vi "FPGA_balancing_noGPS.vi"() -> ()   [LabVIEW 2019]
uses:
  <vilib>/rvi/Emulation/niFpgaGetClockAttributes.vi
  <vilib>/rvi/Emulation/niFpgaSctlEmulationGetInTimedLoop.vi
  <vilib>/rvi/Emulation/niFpgaEmulationReportErrorSimple.vi
  <vilib>/rvi/eio/common/nirviEmuTemplateMethod_errors.vi
  <vilib>/rvi/Emulation/niFpgaCriticalErrorInLSC.vi
  Sub VIs/GlobalVariables.vi
  <vilib>/rvi/Emulation/niFpgaProcessEmulError.vi
  <vilib>/eio/EIONode/EIONode.xnode
  Sub VIs/GPS/UART 8N1/UART 8N1 (FPGA).lvlib
panel:
  out "ESTOP":bool
  in  "Hall Edge Detection":enum16{"falling", "rising"}(ring)
  out "Steering Current":u16
  in  "Steering Enable":bool
  out "SPI Read Acc Data":u8[](array[numeric])
  out "SPI Read Gyro Data":u8[](array[numeric])
  out "Encoder Counts":i32
  in  "Encoder Position Reset":bool
  out "Hall Period (uSec/pulse)":u32
  in  "Steering PWM Frequency":sgl
  in  "Steering PWM Duty Cycle":sgl
  in  "Write Data":u8[](array[numeric])=[0, 0, 0, 0, 0, 0, 0, 0, 0, 0, 0, 0, 0, 0, 0, 0, 0, 0, 0, 0, 0, 0, 0, 0, 0]
  in  "Write":bool
  # "IMU"
  # "Steering motor"
  # "GPS"
  # "Hall sensor"
  # "Encoder"
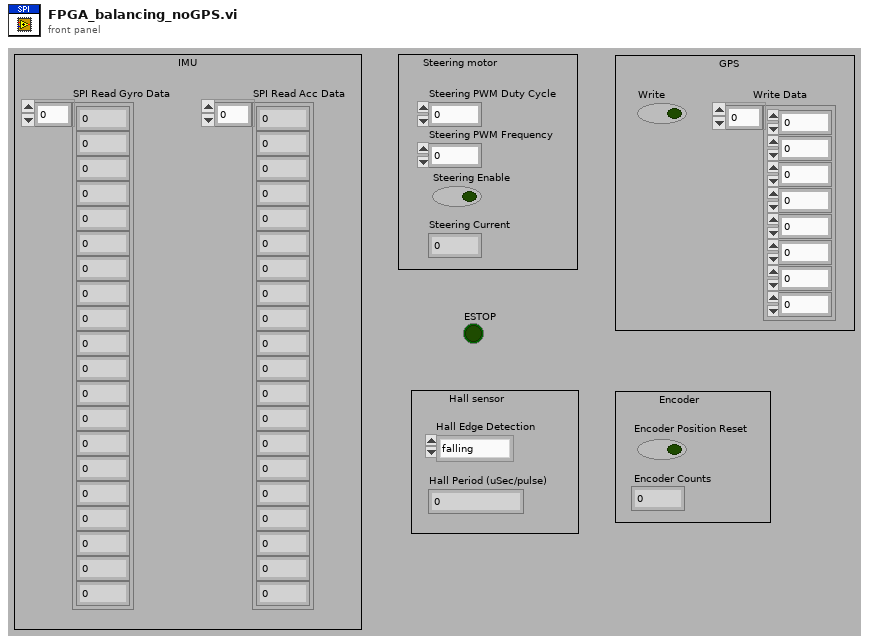
[diagram p1: front panel]
types:
  T1 = cluster{"SCLK":refnum<k21>, "CS":refnum<k21>, "MOSI":refnum<k21>, "MISO":refnum<k21>}
  T2 = typedef "UART 8N1 (FPGA).lvlib/UART Ref.ctl" = cluster{"FPGA I/O":refnum<k21>, "Buffer Ref":refnum<k21>, "Stop Ref":refnum<k21>}
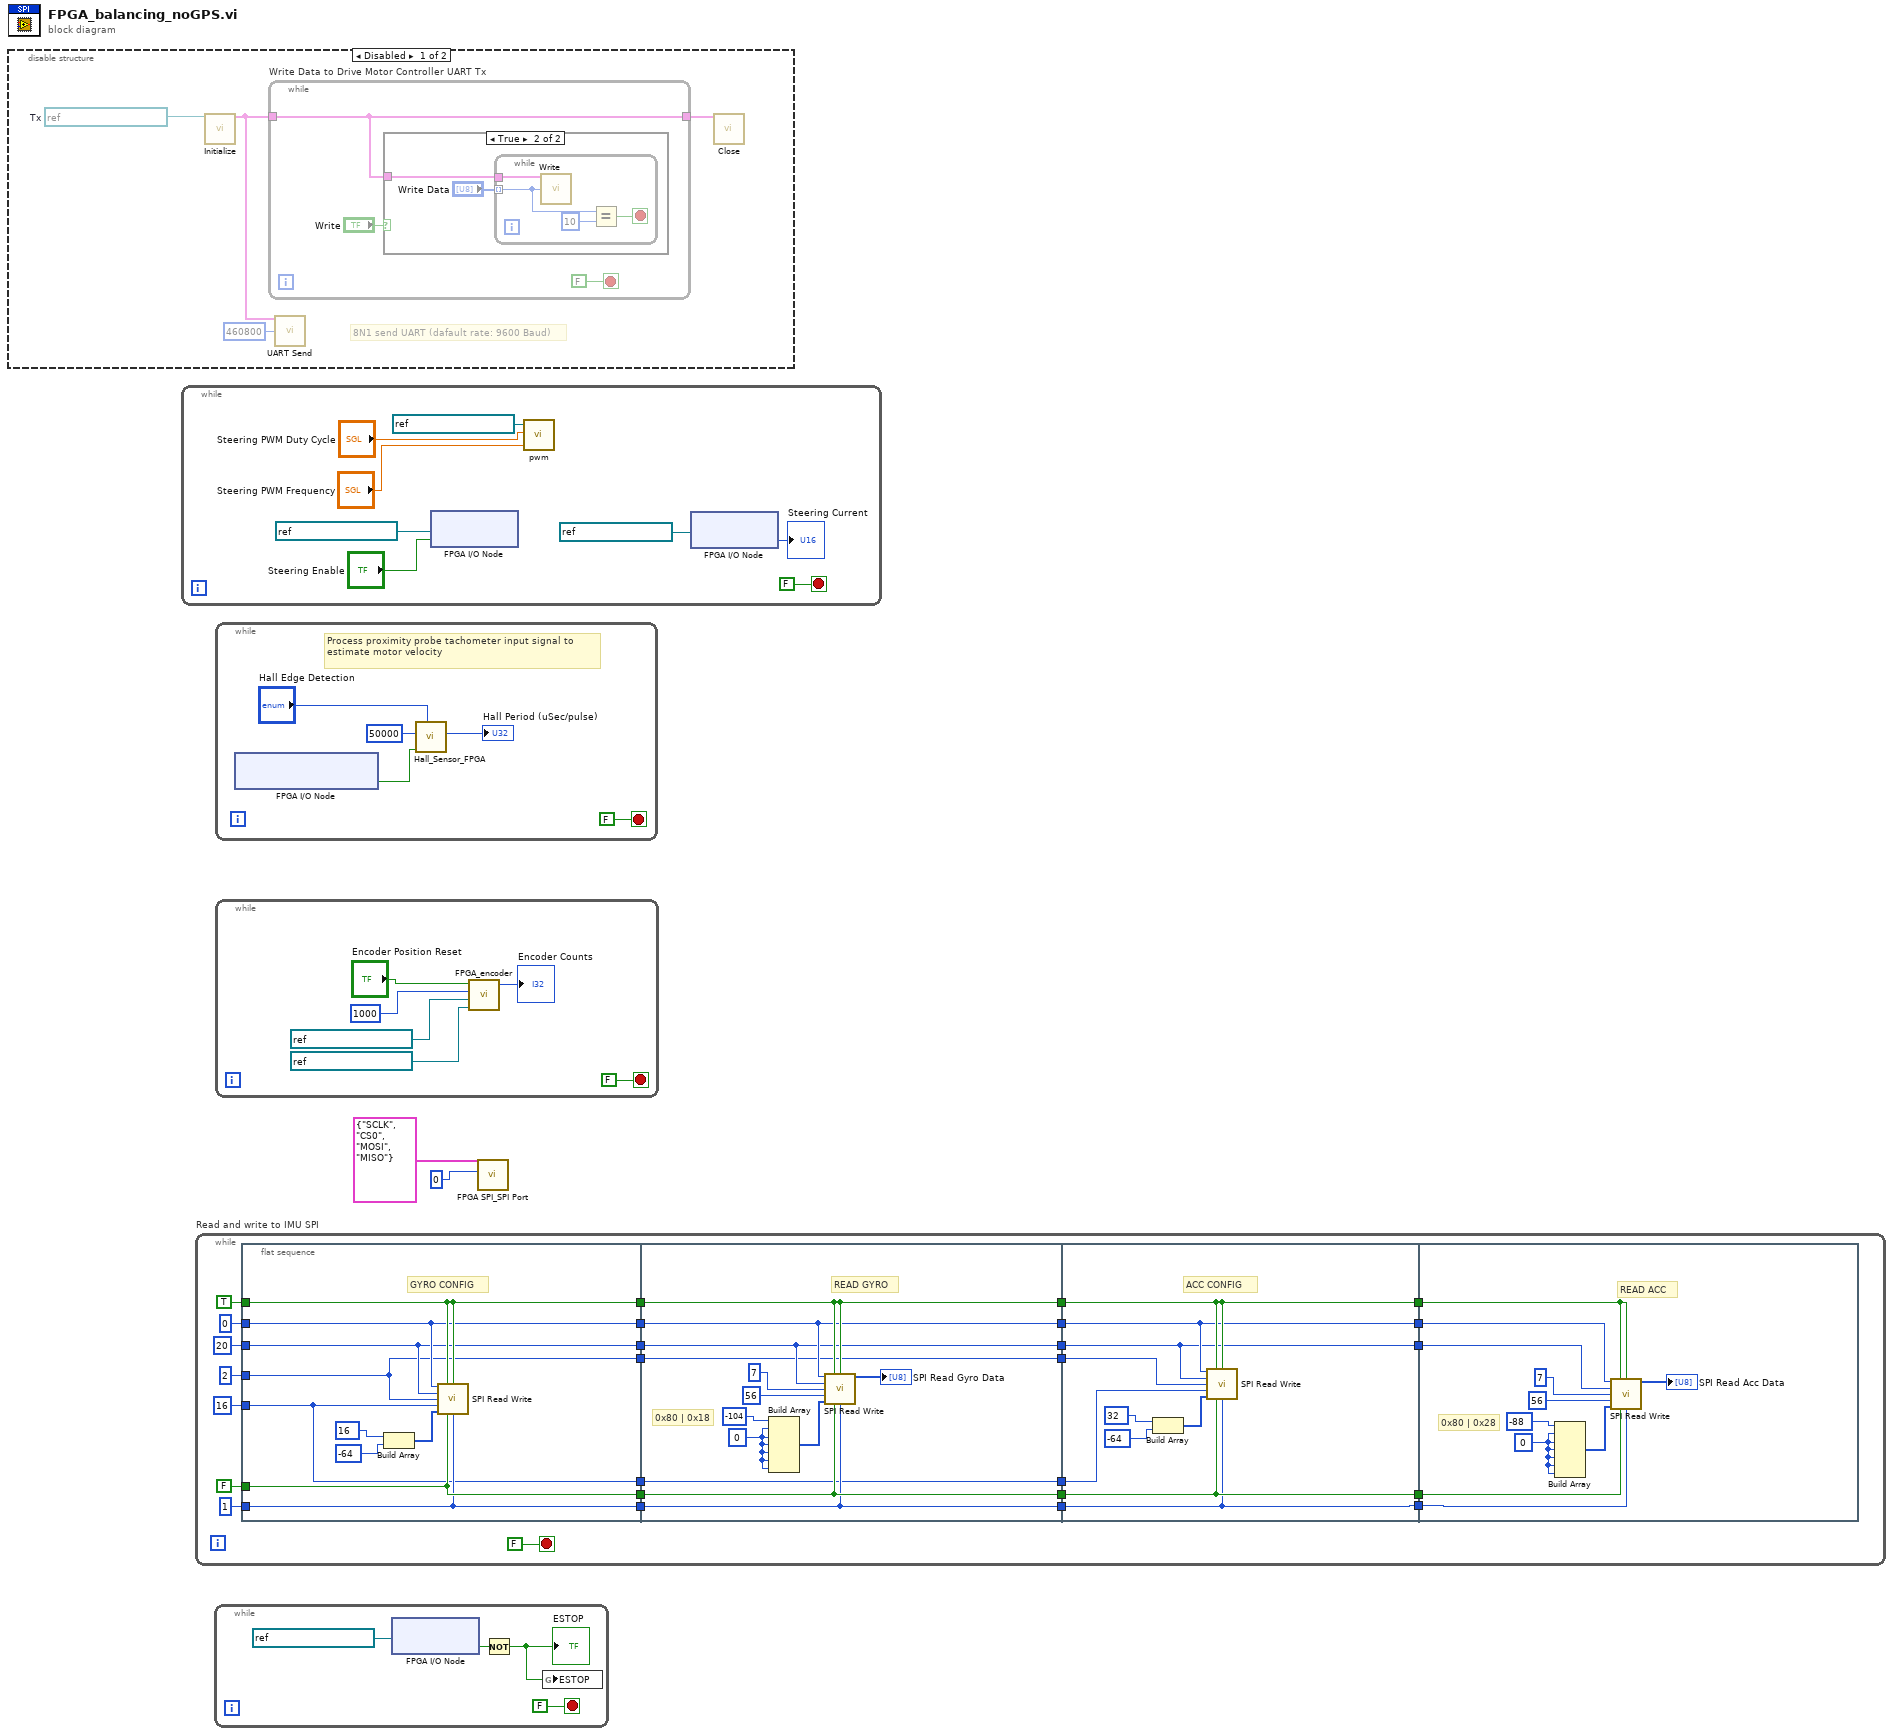
[diagram p0: block diagram]
diagram:
  n1 = disable-structure shown="Disabled" {
    frame Disabled {
      w6 = refnum<k21> "ConnectorA/DIO1"  # Tx
      # "8N1 send UART (dafault rate: 9600 Baud)"
      n2 = call "Initialize.vi"("FPGA I/O"=w6) -> ("BPT Ref"=w5:T2)  [unwired: 14 in]
      n3 = while "Write Data to Drive Motor Controller UART Tx" {
        tunnel: w5 -> [w8]
        tunnel: [w8] -> w4
        stop <- FALSE stop-if-true
        n4 = case "Write" shown="True" "Write" {
          tunnel: w8 -> [_ w11]
          frame False {
          }
          frame True {
            n5 = while {
              tunnel: w11 -> [w15]
              tunnel: "Write Data" -> [w13] mode=indexing
              stop <- w14 stop-if-true
              n6 = call "Write.vi"("UART Ref In"=w15, "Data"=w13) -> ()  [unwired: 12 in, 2 out]
              n7 = Equal?(x=w13, y=u8 10) -> (x = y?=w14:bool)
            }
          }
        }
      }
      n8 = call "UART Send.vi"("UART Ref In"=w5, "Baud Rate (9600)"=u32 460800) -> ()  [unwired: 14 in]
      n9 = call "Close.vi"("UART Ref"=w4) -> ()  [unwired: 15 in]
    }
    frame Enabled {
    }
  }
  n10 = while {
    stop <- FALSE stop-if-true
    n11 = xnode "FPGA I/O Node"("I/O Item"="Steering Enable", "FPGA I/O In"=refnum<k21> "ConnectorB/DIO2") -> ()  [unwired: 1 out]
    n12 = call "pwm.vi"("Frequency (Hz)"="Steering PWM Frequency", "Duty Cycle (%)"="Steering PWM Duty Cycle", "FPGA I/O In"=refnum<k21> "ConnectorB/DIO1") -> ()  [unwired: 1 in]
    n13 = xnode "FPGA I/O Node"("FPGA I/O In"=refnum<k21> "ConnectorB/AI0") -> ("I/O Item"=→"Steering Current":u16)  [unwired: 1 out]
  }
  n14 = while "Read and write to IMU SPI" {
    stop <- FALSE stop-if-true
    n15 = flat-sequence {
      tunnel: u8 1 ("SPI_CS") -> [w53]
      tunnel: TRUE ("SPI_CPOL") -> [w57]
      tunnel: i8 0 ("SPI_Port") -> [w56]
      tunnel: u32 20 ("SPI_Clock Divider") -> [w55]
      tunnel: u16 2 ("SPI_Total Bytes") -> [w51]
      tunnel: u16 16 ("SPI_Total Bits") -> [w52]
      tunnel: FALSE ("SPI_CS Active State") -> [w54]
      tunnel: [w57] -> w36
      tunnel: [w56] -> w35
      tunnel: [w55] -> w34
      tunnel: [w54] -> w28
      tunnel: [w53] -> w27
      tunnel: [w52] -> w26
      tunnel: [w51] -> w25
      tunnel: [w64] -> w50
      tunnel: [w63] -> w49
      tunnel: [w62] -> w48
      tunnel: [w67] -> w47
      tunnel: [w66] -> w46
      tunnel: [w65] -> w45
      tunnel: [w61] -> w44
      tunnel: w36 -> [w67]
      tunnel: w35 -> [w66]
      tunnel: w34 -> [w65]
      tunnel: w28 -> [w64]
      tunnel: w27 -> [w63]
      tunnel: w26 -> [w62]
      tunnel: w25 -> [w61]
      tunnel: w50 -> [w75]
      tunnel: w49 -> [w74]
      tunnel: w48 -> [w79]
      tunnel: w47 -> [w78]
      tunnel: w46 -> [w77]
      tunnel: w45 -> [w76]
      tunnel: w44 -> [w80]
      tunnel: [w78] -> w33
      tunnel: [w77] -> w32
      tunnel: [w76] -> w31
      tunnel: [w75] -> w30
      tunnel: [w74] -> w29
      tunnel: w33 -> [w88]
      tunnel: w32 -> [w87]
      tunnel: w31 -> [w86]
      tunnel: w30 -> [w85]
      tunnel: w29 -> [w84]
      frame #0 {
        # "GYRO CONFIG"
        n16 = Build Array(i8 16 ("Port"), i8 -64 ("Port")) -> (w58:i8[])
        n17 = call "SPI Read Write.vi"("SPI_Port"=w56, "SPI_CPOL"=w57, "SPI_CPHA"=w57, "SPI_Clock Divider"=w55, "SPI_Total Bytes"=w51, "SPI_Total Bits"=w52, "SPI_Write Data"=w58, "SPI_CS Active State"=w54, "SPI_CS"=w53) -> ()  [unwired: 6 in, 1 out]
      }
      frame #1 {
        w72 = i8 0 ("Port")
        # "0x80 | 0x18"
        # "READ GYRO"
        n18 = Build Array(i8 -104 ("Port"), w72, w72, w72, w72, w72, w72) -> (w73:i8[])
        n19 = call "SPI Read Write.vi"("SPI_Port"=w66, "SPI_CPOL"=w67, "SPI_CPHA"=w67, "SPI_Clock Divider"=w65, "SPI_Total Bytes"=u16 7, "SPI_Total Bits"=u16 56, "SPI_Write Data"=w73, "SPI_CS Active State"=w64, "SPI_CS"=w63) -> ("SPI_Read Data"=→"SPI Read Gyro Data":u8[])  [unwired: 6 in]
      }
      frame #2 {
        # "ACC CONFIG"
        n20 = Build Array(i8 32 ("Port"), i8 -64 ("Port")) -> (w81:i8[])
        n21 = call "SPI Read Write.vi"("SPI_Port"=w77, "SPI_CPOL"=w78, "SPI_CPHA"=w78, "SPI_Clock Divider"=w76, "SPI_Total Bytes"=w80, "SPI_Total Bits"=w79, "SPI_Write Data"=w81, "SPI_CS Active State"=w75, "SPI_CS"=w74) -> ()  [unwired: 6 in, 1 out]
      }
      frame #3 {
        w91 = i8 0 ("Port")
        # "0x80 | 0x28"
        # "READ ACC"
        n22 = Build Array(i8 -88 ("Port"), w91, w91, w91, w91, w91, w91) -> (w90:i8[])
        n23 = call "SPI Read Write.vi"("SPI_Port"=w87, "SPI_CPOL"=w88, "SPI_CPHA"=w88, "SPI_Clock Divider"=w86, "SPI_Total Bytes"=u16 7, "SPI_Total Bits"=u16 56, "SPI_Write Data"=w90, "SPI_CS Active State"=w85, "SPI_CS"=w84) -> ("SPI_Read Data"=→"SPI Read Acc Data":u8[])  [unwired: 6 in]
      }
    }
  }
  n24 = while {
    stop <- FALSE stop-if-true
    n25 = xnode "FPGA I/O Node"("FPGA I/O In"=refnum<k21> "ConnectorB/DIO3") -> ("I/O Item"=w95:bool)  [unwired: 1 out]
    n26 = Not(x=w95) -> (.not. x?=w96:bool)
    "ESTOP" <- w96
    n27 = global write "GlobalVariables.vi" "ESTOP"(w96) -> ()
  }
  n28 = while {
    stop <- FALSE stop-if-true
    # "Process proximity probe tachometer input signal to estimate motor velocity"
    n29 = xnode "FPGA I/O Node"() -> ("ConnectorB/DIO10"=w102:bool)  [unwired: 1 in, 1 out]
    n30 = call "Hall_Sensor_FPGA.vi"("Slope"="Hall Edge Detection", "Hall Sensor"=w102, "Bounce time (uSec)"=u32 50000) -> ("Tach Period (uSec/pulse)"=→"Hall Period (uSec/pulse)":u32)  [unwired: 7 in, 1 out]
  }
  n31 = while {
    stop <- FALSE stop-if-true
    n32 = call "FPGA_encoder.vi"("Encoder Channel B"=refnum<k21> "ConnectorB/DIO9", "Encoder Channel A"=refnum<k21> "ConnectorB/DIO8", "Velocity Interval (uSec)"=u32 1000, "Position Reset"="Encoder Position Reset") -> ("Position (Counts)"=→"Encoder Counts":i32)  [unwired: 2 out]
  }
  n33 = call "FPGA SPI_SPI Port.vi"("Port"=i8 0, "FPGA IO"=T1 {"SCLK"="SCLK", "CS"="CS0", "MOSI"="MOSI", "MISO"="MISO"}) -> ()  [unwired: 10 out]
